vi "Set Strings from Ref.vi"(8 "error in (no error)":errorcluster, 9 "Language Index (0)":i32, 10 "GObj Refnum":refnum<vi>, 11 "Control in":refnum<class "Control.lvclass">) -> (0 "error out":errorcluster, 3 "Control out":refnum<class "Control.lvclass">)   [LabVIEW 2013, in "SET Project Data.lvlib" / "Control.lvclass"]
uses:
  Control.lvclass
  GObject/GObject.lvclass
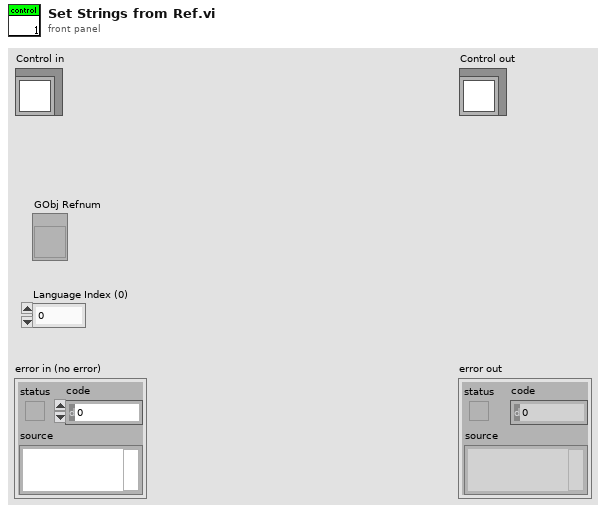
[diagram p1: front panel]
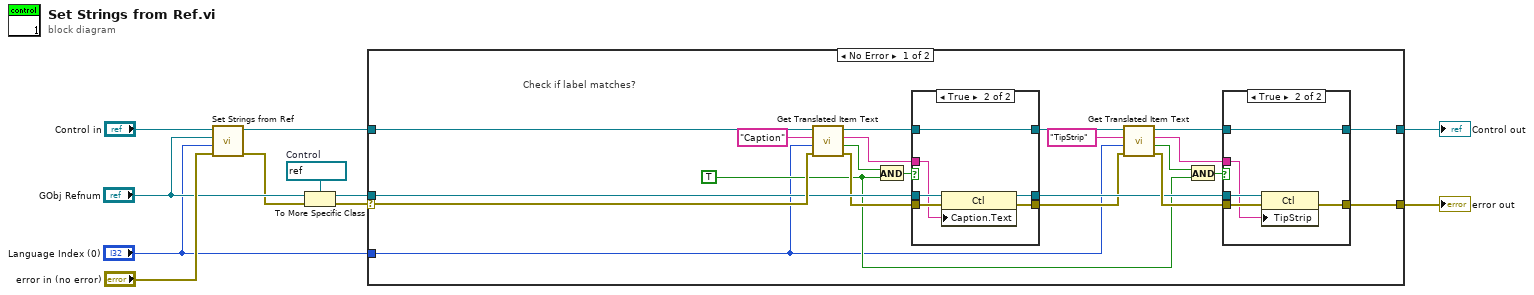
[diagram p0: block diagram]
diagram:
  w8 = refnum<vi> refnum  # Control
  n1 = call-parent "Set Strings from Ref.vi"("error in (no error)"="error in (no error)", "Language Index (0)"="Language Index (0)", "GObj Refnum"="GObj Refnum", "GObject in"="Control in") -> ("error out"=w7:errorcluster, "GObject out"=w4:refnum<class "Control.lvclass">)  [unwired: 6 in]
  n2 = To More Specific Class(target class=w8, reference="GObj Refnum", error in=w7) -> (specific class reference=w5:refnum<vi>, error out=w6:errorcluster)
  n3 = case shown="No Error" w6 {
    selector: w6 -> [w31 w50]
    tunnel: w5 -> [w26 _]
    tunnel: w4 -> [w32 w51]
    tunnel: "Language Index (0)" -> [w12 _]
    tunnel: [w18 w51] -> w2
    tunnel: [w17 w50] -> w1
    frame No Error {
      w13 = TRUE
      # "Check if label matches?"
      n4 = call "Get Translated Item Text.vi"("error in (no error)"=w31, "LangIndex (0)"=w12, "ItemName"="Caption", "GObject in"=w32) -> ("error out"=w25:errorcluster, "Found?"=w29:bool, "Translated Text (ASCII)"=w28:string, "GObject out"=w27:refnum<class "Control.lvclass">)  [unwired: 4 in]
      n5 = And(x=w29, y=w13) -> (x .and. y?=w30:bool)
      n6 = case shown="True" w30 {
        tunnel: w28 -> [_ w47]
        tunnel: w27 -> [w43 w46]
        tunnel: w26 -> [w41 w49]
        tunnel: w25 -> [w42 w48]
        tunnel: [w43 w46] -> w16
        tunnel: [w42 w45] -> w14
        tunnel: [w41 w44] -> w15
        frame False {
        }
        frame True {
          n7 = property class="Ctl"(reference=w49, error in=w48, "Caption.Text"=w47) -> (reference out=w44:refnum<vi>, error out=w45:errorcluster)
        }
      }
      n8 = call "Get Translated Item Text.vi"("error in (no error)"=w14, "LangIndex (0)"=w12, "ItemName"="TipStrip", "GObject in"=w16) -> ("error out"=w24:errorcluster, "Found?"=w21:bool, "Translated Text (ASCII)"=w22:string, "GObject out"=w23:refnum<class "Control.lvclass">)  [unwired: 4 in]
      n9 = And(x=w21, y=w13) -> (x .and. y?=w20:bool)
      n10 = case shown="True" w20 {
        tunnel: w22 -> [_ w38]
        tunnel: w23 -> [w35 w37]
        tunnel: w15 -> [_ w40]
        tunnel: w24 -> [w34 w39]
        tunnel: [w35 w37] -> w18
        tunnel: [w34 w36] -> w17
        frame False {
        }
        frame True {
          n11 = property class="Ctl"(reference=w40, error in=w39, "TipStrip"=w38) -> (error out=w36:errorcluster)  [unwired: 1 out]
        }
      }
    }
    frame Error {
    }
  }
  "error out" <- w1
  "Control out" <- w2
